vi "Individual curve visualization-HY.vi"() -> ()   [LabVIEW 2016]
panel:
  in  "Tab Control":enum32{"Drag R and 4T R", " Line cut"}(tab)=enum." Line cut"
  in  "Input figure":cluster{dbl[], dbl[]}[](graph)
  out "Mean vs Curve":cluster{dbl[], dbl[]}(graph)
  in  "Group #":i32=40
  in  "Auto moving cursor X ?":bool
  in  "Wait time X":dbl
  in  "Auto moving cursor Y ?":bool
  in  "Wait time Y":dbl
  in  "Drag V from V2":dbl[][](graph)=array4000x21[84000 elements]
  out "Trans R":cluster{dbl[], "Drag V from V2":dbl[]}(graph)
  out "Idrive":cluster{dbl[], dbl[]}[](graph)
  in  "stop Auto X":bool
  in  "stop Auto Y":bool
  in  "stop":bool
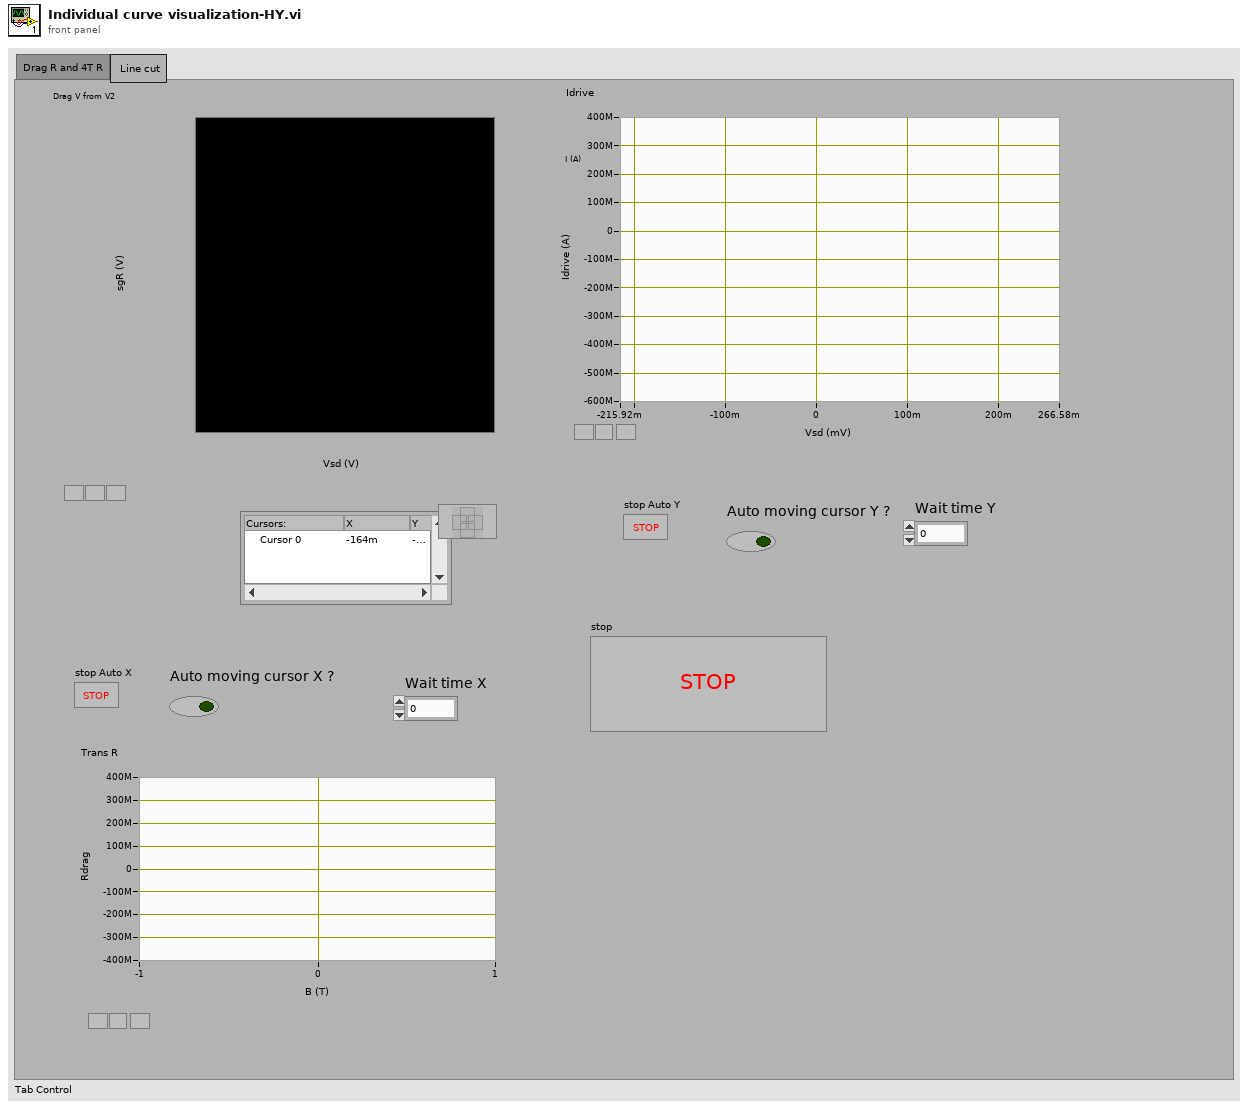
[diagram p1: front panel]
types:
  T1 = typedef "LVOffsetAndMultiplierTypeDef.ctl" = cluster{"Offset":dbl, "Multiplier":dbl}
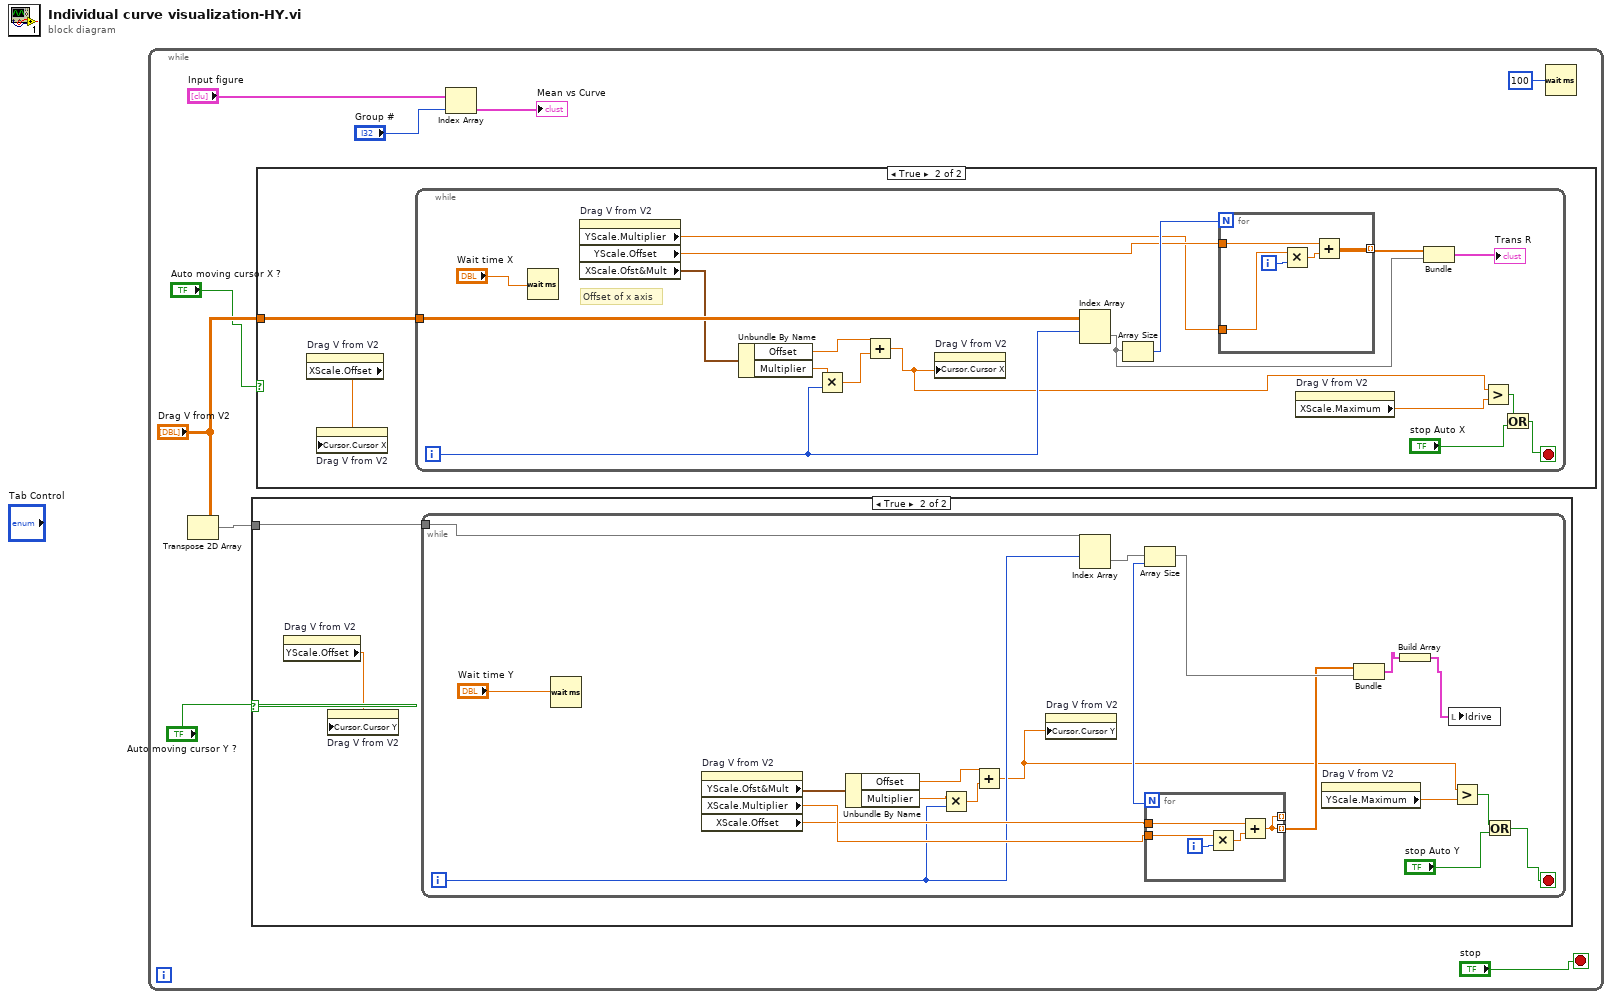
[diagram p0: block diagram]
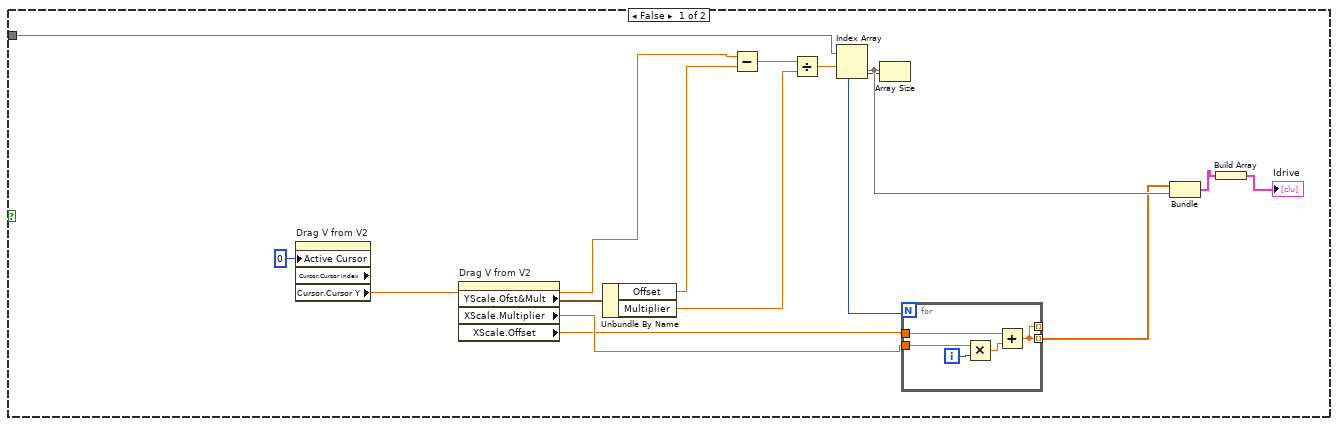
[diagram p2: hidden frame]
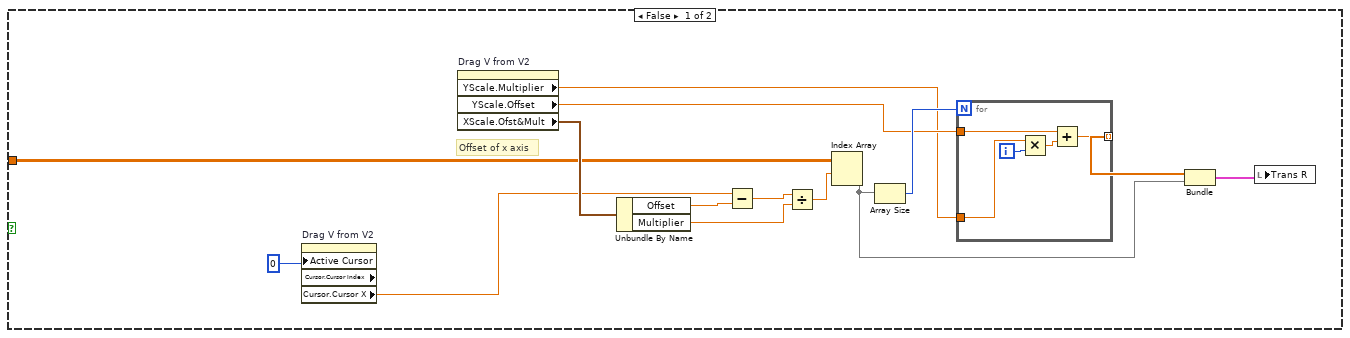
[diagram p3: hidden frame]
diagram:
  n1 = while {
    stop <- "stop" stop-if-true
    n2 = Transpose 2D Array(2D array="Drag V from V2") -> (transposed array=w7:dbl[][])
    n3 = case shown="True" "Auto moving cursor Y ?" {
      tunnel: w7 -> [w24 w31]
      frame False {
        n4 = property on="Drag V from V2" class="IntGraph (strict)" props=["Active Cursor", "Cursor", "Cursor Index", "Cursor", "Cursor Y"]("Active Cursor"=u32 0) -> ("Cursor.Cursor Y"=w12:dbl)  [unwired: 2 in, 3 out]
        n5 = property on="Drag V from V2" class="IntGraph (strict)"() -> ("YScale.Ofst&Mult"=w23:T1, "XScale.Multiplier"=w11:dbl, "XScale.Offset"=w10:dbl)  [unwired: 2 in, 2 out]
        n6 = Unbundle By Name(w23) -> ("Offset"=w20:dbl, "Multiplier"=w21:dbl)
        n7 = Subtract(x=w12, y=w20) -> (x-y=w22:dbl)
        n8 = Divide(x=w22, y=w21) -> (x/y=w16:dbl)
        n9 = Index Array(array=w24, index (row)=w16) -> (element=w19:dbl[])  [unwired: 1 in]
        n10 = Array Size(array=w19) -> (size(s)=w18:i32)
        n11 = for {
          N: w18 -> [_]
          tunnel: w11 -> [w28]
          tunnel: w10 -> [w26]
          tunnel: [w25] -> _ mode=indexing
          tunnel: [w25] -> w17 mode=indexing
          i -> [w29]
          n12 = Multiply(x=w28, y=w29) -> (x*y=w27:dbl)
          n13 = Add(x=w26, y=w27) -> (x+y=w25:dbl)
        }
        n14 = Bundle(w17, w19) -> (w15:cluster{dbl[], dbl[]})  [unwired: 1 in]
        n15 = Build Array(w15) -> (→"Idrive":cluster{dbl[], dbl[]}[])
      }
      frame True {
        n16 = property on="Drag V from V2" class="IntGraph (strict)"() -> ("YScale.Offset"=w30:dbl)  [unwired: 2 in, 2 out]
        n17 = property on="Drag V from V2" class="IntGraph (strict)"("Cursor.Cursor Y"=w30) -> ()  [unwired: 2 in, 2 out]
        n18 = while {
          tunnel: w31 -> [w50]
          i -> [w39]
          stop <- w32 stop-if-true
          n19 = Wait (ms)(milliseconds to wait="Wait time Y") -> ()  [unwired: 1 out]
          n20 = property on="Drag V from V2" class="IntGraph (strict)"() -> ("YScale.Ofst&Mult"=w49:T1, "XScale.Multiplier"=w44:dbl, "XScale.Offset"=w43:dbl)  [unwired: 2 in, 2 out]
          n21 = Unbundle By Name(w49) -> ("Offset"=w38:dbl, "Multiplier"=w40:dbl)
          n22 = Multiply(x=w40, y=w39) -> (x*y=w37:dbl)
          n23 = Add(x=w38, y=w37) -> (x+y=w36:dbl)
          n24 = property on="Drag V from V2" class="IntGraph (strict)"("Cursor.Cursor Y"=w36) -> ()  [unwired: 2 in, 2 out]
          n25 = Index Array(array=w50, index (row)=w39) -> (element=w48:dbl[])  [unwired: 1 in]
          n26 = Array Size(array=w48) -> (size(s)=w47:i32)
          n27 = for {
            N: w47 -> [_]
            tunnel: w44 -> [w54]
            tunnel: w43 -> [w52]
            tunnel: [w51] -> _ mode=indexing
            tunnel: [w51] -> w46 mode=indexing
            i -> [w55]
            n28 = Multiply(x=w54, y=w55) -> (x*y=w53:dbl)
            n29 = Add(x=w52, y=w53) -> (x+y=w51:dbl)
          }
          n30 = property on="Drag V from V2" class="IntGraph (strict)"() -> ("YScale.Maximum"=w35:dbl)  [unwired: 2 in, 2 out]
          n31 = Bundle(w46, w48) -> (w45:cluster{dbl[], dbl[]})  [unwired: 1 in]
          n32 = Build Array(w45) -> (w42:cluster{dbl[], dbl[]}[])
          n33 = local write "Idrive"(w42) -> ()
          n34 = Greater?(x=w36, y=w35) -> (0:w34:bool)
          n35 = Or(x=w34, y="stop Auto Y") -> (x .or. y?=w32:bool)
        }
      }
    }
    n36 = case shown="True" "Auto moving cursor X ?" {
      tunnel: "Drag V from V2" -> [w62 w76]
      frame False {
        # "Offset of x axis"
        n37 = property on="Drag V from V2" class="IntGraph (strict)" props=["Active Cursor", "Cursor", "Cursor Index", "Cursor", "Cursor X"]("Active Cursor"=u32 0) -> ("Cursor.Cursor X"=w60:dbl)  [unwired: 2 in, 3 out]
        n38 = property on="Drag V from V2" class="IntGraph (strict)"() -> ("YScale.Multiplier"=w58:dbl, "YScale.Offset"=w59:dbl, "XScale.Ofst&Mult"=w69:T1)  [unwired: 2 in, 2 out]
        n39 = Unbundle By Name(w69) -> ("Offset"=w63:dbl, "Multiplier"=w64:dbl)
        n40 = Subtract(x=w60, y=w63) -> (x-y=w68:dbl)
        n41 = Divide(x=w68, y=w64) -> (x/y=w61:dbl)
        n42 = Index Array(array=w62, index (row)=w61) -> (element=w66:dbl[])  [unwired: 1 in]
        n43 = Array Size(array=w66) -> (size(s)=w67:i32)
        n44 = for {
          N: w67 -> [_]
          tunnel: w58 -> [w73]
          tunnel: w59 -> [w71]
          tunnel: [w70] -> w65 mode=indexing
          i -> [w74]
          n45 = Multiply(x=w73, y=w74) -> (x*y=w72:dbl)
          n46 = Add(x=w71, y=w72) -> (x+y=w70:dbl)
        }
        n47 = Bundle(w65, "Drag V from V2"=w66) -> (w56:cluster{dbl[], "Drag V from V2":dbl[]})  [unwired: 1 in]
        n48 = local write "Trans R"(w56) -> ()
      }
      frame True {
        n49 = property on="Drag V from V2" class="IntGraph (strict)"() -> ("XScale.Offset"=w75:dbl)  [unwired: 2 in, 2 out]
        n50 = property on="Drag V from V2" class="IntGraph (strict)"("Cursor.Cursor X"=w75) -> ()  [unwired: 2 in, 2 out]
        n51 = while {
          tunnel: w76 -> [w91]
          i -> [w85]
          stop <- w77 stop-if-true
          # "Offset of x axis"
          n52 = Wait (ms)(milliseconds to wait="Wait time X") -> ()  [unwired: 1 out]
          n53 = property on="Drag V from V2" class="IntGraph (strict)"() -> ("YScale.Multiplier"=w89:dbl, "YScale.Offset"=w90:dbl, "XScale.Ofst&Mult"=w87:T1)  [unwired: 2 in, 2 out]
          n54 = Unbundle By Name(w87) -> ("Offset"=w84:dbl, "Multiplier"=w86:dbl)
          n55 = Multiply(x=w86, y=w85) -> (x*y=w83:dbl)
          n56 = Add(x=w84, y=w83) -> (x+y=w81:dbl)
          n57 = property on="Drag V from V2" class="IntGraph (strict)"("Cursor.Cursor X"=w81) -> ()  [unwired: 2 in, 2 out]
          n58 = Index Array(array=w91, index (row)=w85) -> (element=w93:dbl[])  [unwired: 1 in]
          n59 = Array Size(array=w93) -> (size(s)=w94:i32)
          n60 = for {
            N: w94 -> [_]
            tunnel: w89 -> [w98]
            tunnel: w90 -> [w96]
            tunnel: [w95] -> w92 mode=indexing
            i -> [w99]
            n61 = Multiply(x=w98, y=w99) -> (x*y=w97:dbl)
            n62 = Add(x=w96, y=w97) -> (x+y=w95:dbl)
          }
          n63 = property on="Drag V from V2" class="IntGraph (strict)"() -> ("XScale.Maximum"=w80:dbl)  [unwired: 2 in, 2 out]
          n64 = Bundle(w92, "Drag V from V2"=w93) -> (→"Trans R":cluster{dbl[], "Drag V from V2":dbl[]})  [unwired: 1 in]
          n65 = Greater?(x=w81, y=w80) -> (0:w79:bool)
          n66 = Or(x=w79, y="stop Auto X") -> (x .or. y?=w77:bool)
        }
      }
    }
    n67 = Index Array(array="Input figure", index="Group #") -> (element=→"Mean vs Curve":cluster{dbl[], dbl[]})
    n68 = Wait (ms)(milliseconds to wait=u32 100) -> ()  [unwired: 1 out]
  }
